vi "Set Meta Data.vi"(7 "Tree ID":string, 8 "Error In":errorcluster, 10 "Meta Data":string, 11 "Tree Manager":T1) -> (0 "Error Out":errorcluster, 3 "Tree Manager":T1)   [LabVIEW 2020, in "NI_VIAnCFGDataStructure.lvlib" / "Tree.lvclass"]
doc: "Set the Meta Data of the Tree."
uses:
  <vilib>/addons/analyzer/VIAnCFGDataStructure/Tree Manager/Tree.lvclass
  <vilib>/addons/analyzer/VIAnCFGDataStructure/Tree Manager/Typedefs/Session Handle.ctl
  <vilib>/addons/analyzer/VIAnCFGDataStructure/Tree Manager/Tree.lvclass/Tree.ctl
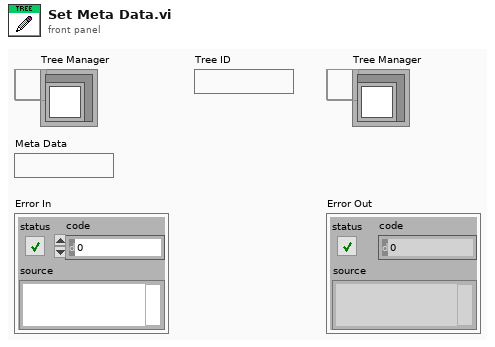
[diagram p1: front panel]
types:
  T1 = typedef "NI_VIAnCFGDataStructure.lvlib/Tree.lvclass/Session Handle.ctl" = refnum<data-value>
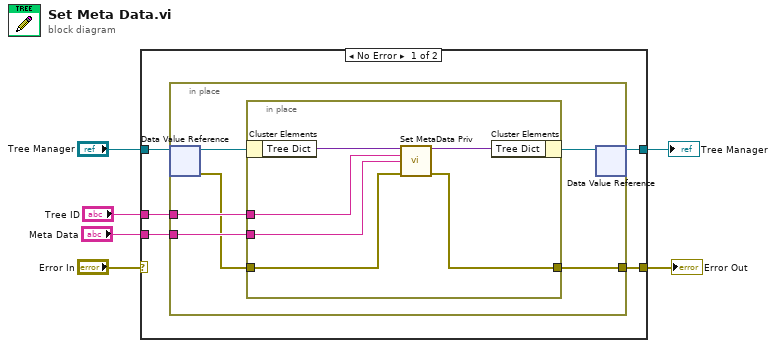
[diagram p0: block diagram]
diagram:
  n1 = case shown="No Error" "Error In" {
    selector: "Error In" -> [_ w24]
    tunnel: "Tree Manager" -> [w11 w25]
    tunnel: [w10 w25] -> w5
    tunnel: [w9 w24] -> w3
    tunnel: "Tree ID" -> [w8 _]
    tunnel: "Meta Data" -> [w7 _]
    frame No Error {
      n2 = in-place {
        in-place-border: [w16] -> w9
        in-place-border: w8 -> [w14]
        in-place-border: w7 -> [w13]
        n3 = in-place-dvr #1(w11) -> (w17:refnum<class "Tree.lvclass">, w12:errorcluster)
        n4 = in-place {
          in-place-border: [w21] -> w16
          in-place-border: w12 -> [w20]
          in-place-border: w14 -> [w19]
          in-place-border: w13 -> [w18]
          n5 = in-place-cluster #2(w17) -> ("Tree Dict"=w23:variant)
          n6 = call <vilib>:"Set MetaData Priv.vi"("Tree Dict"=w23, "Tree ID"=w19, "MetaData"=w18, "error in"=w20) -> ("Tree Dict"=w22:variant, "error out"=w21:errorcluster)  [unwired: 10 in]
          n7 = in-place-cluster #2("Tree Dict"=w22) -> (w15:refnum<class "Tree.lvclass">)
        }
        n8 = in-place-dvr #1(w15) -> (w10:T1)  [unwired: 1 out]
      }
    }
    frame Error {
    }
  }
  "Tree Manager" <- w5
  "Error Out" <- w3
